vi "AVS_GetOemParameter.vi"(2 "a_pOemData":u8[](array[numeric]), 3 "a_hDevice":i32) -> (0 "a_pOemData":u8[](array[numeric]), 1 "Output Value":i32)   [LabVIEW 2018]
uses:
  avaspecx64.dll
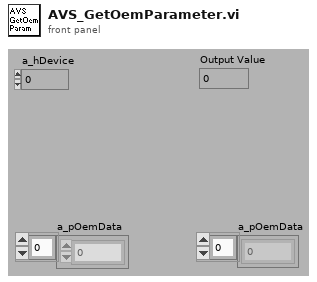
[diagram p1: front panel]
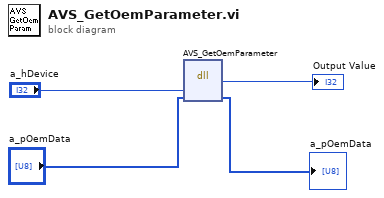
[diagram p0: block diagram]
diagram:
  n1 = dll-call lib="C:/AvaSpecX64-DLL_9.7/examples/LabView/LabViewSingleChan/avaspecx64.dll" fn="AVS_GetOemParameter"("a_hDevice"="a_hDevice", "a_pOemData"="a_pOemData") -> ("return type"=→"Output Value":i32, "a_pOemData"=→"a_pOemData":u8[])  [unwired: 4 in, 2 out]
